vi "UI_recaptionNumerics.vi"(8 "error in (no error)":errorcluster, 10 "Names":string[](array[string]), 11 "Numeric Refs":refnum<vi>[](array[refnum])) -> (0 "error out":errorcluster)   [LabVIEW 2020]
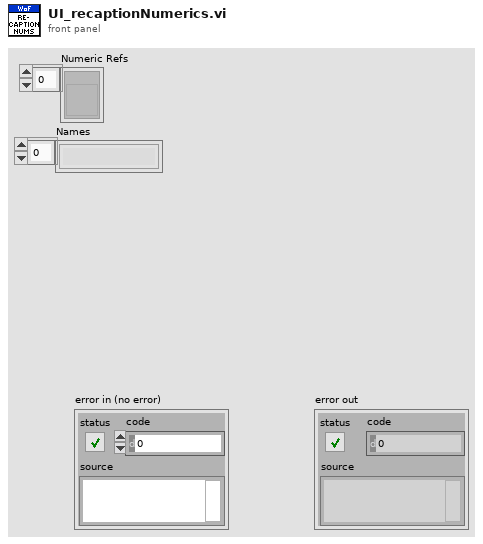
[diagram p1: front panel]
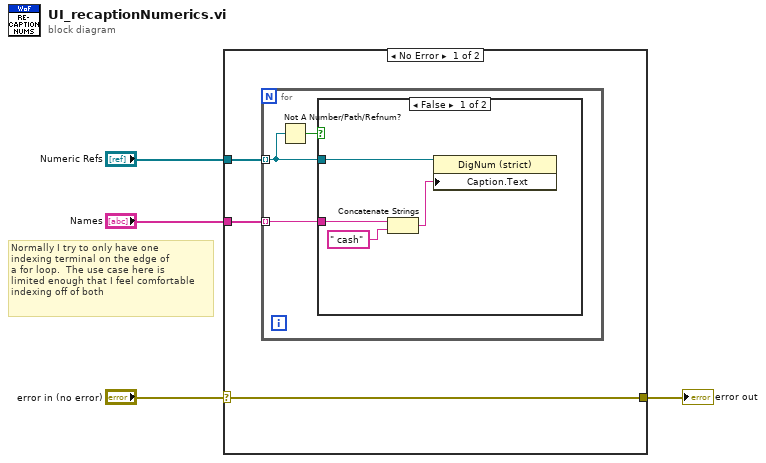
[diagram p0: block diagram]
diagram:
  # "Normally I try to only have one\nindexing terminal on the edge of\na for loop.  The use case here is \nlimited enough that I feel comfortable\nindexing off of both"
  n1 = case shown="No Error" "error in (no error)" {
    selector: "error in (no error)" -> [w5 w15]
    tunnel: "Numeric Refs" -> [w7 _]
    tunnel: "Names" -> [w6 _]
    tunnel: [w5 w15] -> w2
    frame No Error {
      n2 = for {
        tunnel: w7 -> [w8] mode=indexing
        tunnel: w6 -> [w9] mode=indexing
        n3 = Not A Number/Path/Refnum?(number/path/refnum=w8) -> (NaN/Path/Refnum?=w10:bool)
        n4 = case shown="False" w10 {
          tunnel: w9 -> [w13 _]
          tunnel: w8 -> [w14 _]
          frame False {
            n5 = Concatenate Strings(w13, " cash") -> (w11:string)
            n6 = property class="DigNum (strict)"(reference=w14, "Caption.Text"=w11) -> ()  [unwired: 1 in, 2 out]
          }
          frame True {
          }
        }
      }
    }
    frame Error {
    }
  }
  "error out" <- w2
